vi "tsfifo_read_lin_buffer_frame_count.vi"(8 "错误输入（无错误）":errorcluster, 10 "AAppChannel":i32(ring) items=["CHN1", "CHN2", "CHN3", "CHN4", "CHN5", "CHN6", "CHN7", "CHN8", "CHN9", "CHN10", "CHN11", "CHN12", "CHN13", "CHN14", "CHN15", "CHN16", "CHN17", "CHN18", "CHN19", "CHN20", "CHN21", "CHN22", "CHN23", "CHN24", "CHN25", "CHN26", "CHN27", "CHN28", "CHN29", "CHN30", "CHN31", "CHN32"], 11 "路径输入":path) -> (0 "错误输出":errorcluster, 1 "ACount":i32, 2 "return":i32, 3 "路径输出":path)   [LabVIEW 2014]
doc: "Function Introduction :\nRead the number of LIN messages cached in the channel\nCall location :\nIn situations where it is necessary to determine whether there are LIN messages in the cache\ninput parameter :\nAChn: Hardware Channel\nACount: Return count\nReturn value :\nReturn the number of LIN messages in the cache"
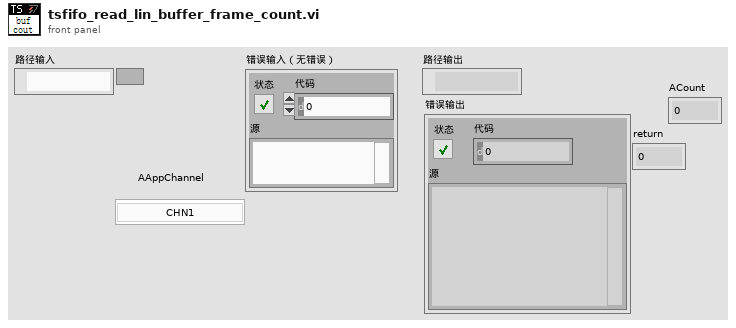
[diagram p1: front panel]
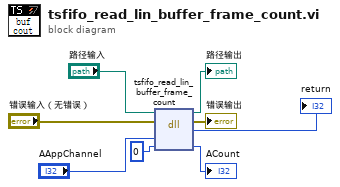
[diagram p0: block diagram]
diagram:
  n1 = dll-call lib="D:/Program Files (x86)/TOSUN/TSMaster/Data/SDK/lib/x86/TSMaster.dll" fn="tsfifo_read_lin_buffer_frame_count"(path in="路径输入", error in="错误输入（无错误）", "AChn"="AAppChannel", "ACount"=0) -> (path out=→"路径输出":path, error out=→"错误输出":errorcluster, "返回类型"=→"return":i32, "ACount"=→"ACount":i32)  [unwired: 2 in]
